vi "Tempcontroll.vi"() -> ()   [LabVIEW 2010]
panel:
  in  "String":string
  in  "mode (0)":i16
  in  "error in":errorcluster
  in  "address string":string="19"
  out "error out":errorcluster
  in  "Spannung in V":dbl=200.0 format="%.2f"
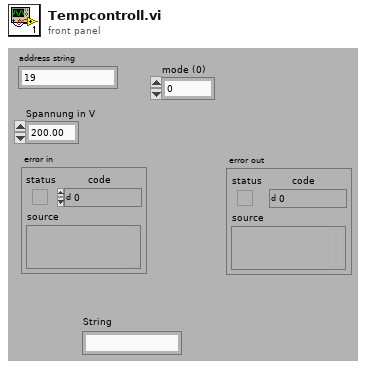
[diagram p1: front panel]
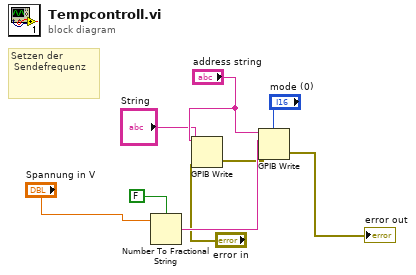
[diagram p0: block diagram]
diagram:
  # "Setzen der \n Sendefrequenz"
  n1 = Number To Fractional String(use system decimal point (T)=FALSE, number="Spannung in V") -> (F-format string=w5:string)  [unwired: 2 in]
  n2 = GPIB Write(0:"address string", 1:"String", 3:"error in") -> (6:w1:errorcluster)  [unwired: 2 in, 1 out]
  n3 = GPIB Write(0:"address string", 1:w5, 2:"mode (0)", 3:w1) -> (6:→"error out":errorcluster)  [unwired: 1 in, 1 out]
